vi "DSDLL Fetch From Digitizing Process.vi"(7 "max wait for packet [ms]":i32=50, 8 "error in":errorcluster, 11 "dsdll in":T3) -> (0 "error out":errorcluster, 1 "auxiliary sampling data":T1, 2 "data block":T2, 3 "dsdll out":T3, 4 "fetching done?":bool)   [LabVIEW 2013, in "DSDLL Virtual Digitizer.lvlib"]
doc: "Tries to fetch data block from digitizing data queue. It waits for predefined amount of time. If fetch timeout is reached it returns no data and no error. If digitizing or fetching timeout is reached it returns timout error. If the last data block was detected it also waits for digitizing process exit. If the process won't return it generates error. If the \ndigitizing process terminates prematurely it will return error. The 'auxiliary sampling data' are valid only if 'valid?' flag in it is True. 'Data block' content is valid only if 'valid?' flag is true. The caller of this VI must collect the data whenever the 'valid?' flag(s) are True. Caller of this VI must always check 'fetching done?' flag and when it is True or function returned error it shall not be called again."
uses:
  DSDLL Virtual Digitizer.lvlib
  DSDLL Session.ctl
  dsdll.lvlibp/dsdll_instance.ctl
  dsdll.lvlibp/dsdll_device_record.ctl
  DSDLL Process Config.ctl
  DSDLL Data Packet.ctl
  DSDLL Aux Record Data.ctl
  <vilib>/Utility/error.llb/Error Cluster From Error Code.vi
  <vilib>/ErrorRing/Error Ring.xnode
  dsdll.lvlibp
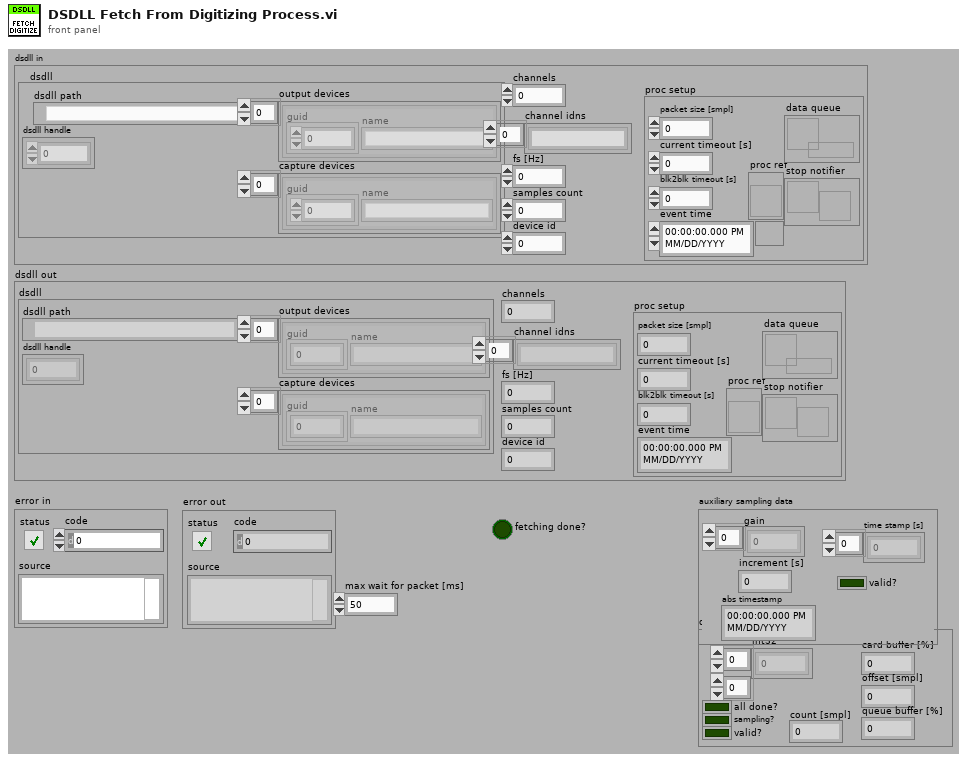
[diagram p1: front panel]
types:
  T1 = typedef "DSDLL Virtual Digitizer.lvlib/DSDLL Aux Record Data.ctl" = cluster{"time stamp [s]":dbl[], "gain":dbl[], "increment [s]":dbl, "valid?":bool, "abs timestamp":timestamp}
  T2 = typedef "DSDLL Virtual Digitizer.lvlib/DSDLL Data Packet.ctl" = cluster{"int32":i32[][], "card buffer [%]":dbl, "all done?":bool, "offset [smpl]":i32, "sampling?":bool, "queue buffer [%]":dbl, "count [smpl]":i32, "valid?":bool}
  T3 = typedef "DSDLL Virtual Digitizer.lvlib/DSDLL Session.ctl" = cluster{"dsdll":T4, "channels":i32, "device id":i32, "channel idns":string[], "proc setup":T6, "samples count":i32, "fs [Hz]":dbl}
  T4 = typedef "dsdll.lvlibp/dsdll_instance.ctl" = cluster{"dsdll path":path, "dsdll handle":u8[], "output devices":T5[], "capture devices":T5[]}
  T5 = typedef "dsdll.lvlibp/dsdll_device_record.ctl" = cluster{"guid":u8[], "name":string}
  T6 = typedef "DSDLL Virtual Digitizer.lvlib/DSDLL Process Config.ctl" = cluster{"packet size [smpl]":i32, "current timeout [s]":dbl, "blk2blk timeout [s]":dbl, "event time":timestamp, "data queue":refnum<queue>, "stop notifier":refnum<notifier>, "proc ref":refnum<vi>}
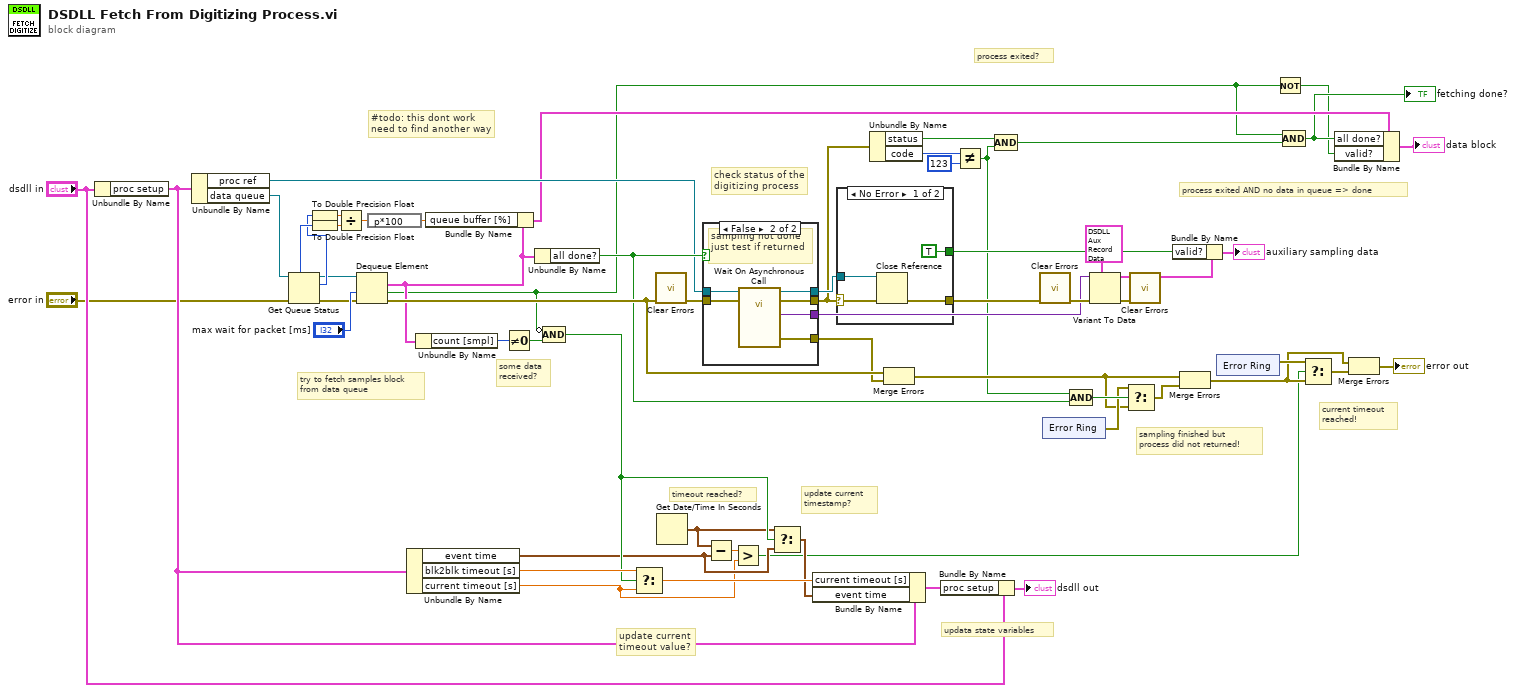
[diagram p0: block diagram]
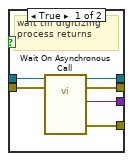
[diagram p3: hidden frame]
diagram:
  # "process exited AND no data in queue => done"
  # "process exited?"
  # "update current\ntimestamp?"
  # "update current \ntimeout value?"
  # "some data\nreceived?"
  # "#todo: this dont work\nneed to find another way"
  # "updata state variables"
  # "check status of the\ndigitizing process"
  # "try to fetch samples block\nfrom data queue"
  # "current timeout\nreached!"
  # "sampling finished but\nprocess did not returned!"
  # "timeout reached?"
  n1 = Unbundle By Name("dsdll in") -> ("proc setup"=w41:T6)
  n2 = Unbundle By Name(w41) -> ("proc ref"=w42:refnum<vi>, "data queue"=w29:refnum<queue>)
  n3 = Get Queue Status(queue=w29, error in (no error)="error in") -> (queue out=w31:refnum<queue>, max queue size=w37:i32, # pending remove=w32:i32, error out=w38:errorcluster)  [unwired: 1 in, 4 out]
  n4 = To Double Precision Float(number=w32) -> (double precision float=w33:dbl)
  n5 = To Double Precision Float(number=w37) -> (double precision float=w34:dbl)
  n6 = Divide(x=w33, y=w34) -> (x/y=w36:dbl)
  n7 = Dequeue Element(queue=w31, timeout in ms (-1)="max wait for packet [ms]", error in (no error)=w38) -> (element=w25:T2, timed out?=w1:bool, error out=w57:errorcluster)  [unwired: 1 out]
  n8 = expression code="p*100"(w36) -> (w35:dbl)
  n9 = Unbundle By Name(w41) -> ("event time"=w19:timestamp, "blk2blk timeout [s]"=w22:dbl, "current timeout [s]"=w3:dbl)
  n10 = Unbundle By Name(w25) -> ("count [smpl]"=w24:i32)
  n11 = Bundle By Name(cluster=w25, "queue buffer [%]"=w35) -> (w26:T2)
  n12 = Not Equal To 0?(x=w24) -> (x != 0?=w23:bool)
  n13 = Unbundle By Name(w25) -> ("all done?"=w49:bool)
  n14 = Compound Arithmetic op=AND(invert w1, w23) -> (w21:bool)
  n15 = Select(t=w22, s=w21, f=w3) -> (s? t:f=w18:dbl)
  n16 = call <vilib>:"Clear Errors.vi"("error in (no error)"=w57) -> ("error out"=w58:errorcluster)  [unwired: 6 in]
  n17 = Get Date/Time In Seconds() -> (seconds since 1Jan1904=w20:timestamp)
  n18 = case shown="False" w49 {
    tunnel: w42 -> [w66 w72]
    tunnel: w58 -> [w65 w71]
    tunnel: [w64 w70] -> w56
    tunnel: [w63 w69] -> w10
    tunnel: [w62 w68] -> w12
    tunnel: [w61 w67] -> w43
    frame True {
      # "wait till digitizing\nprocess returns"
      n19 = call-by-ref "Wait On Asynchronous Call"(reference=w66, error in=w65) -> (reference out=w61:refnum<vi>, error out=w63:errorcluster, 0:"error out"=w64:errorcluster, "auxiliary data out"=w62:variant)  [unwired: 10 in]
    }
    frame False {
      # "sampling not done\njust test if returned"
      n20 = call-by-ref "Wait On Asynchronous Call"(reference=w72, error in=w71) -> (reference out=w67:refnum<vi>, error out=w69:errorcluster, 0:"error out"=w70:errorcluster, "auxiliary data out"=w68:variant)  [unwired: 10 in]
    }
  }
  n21 = Subtract(x=w20, y=w19) -> (x-y=w59:dbl)
  n22 = Greater?(x=w59, y=w3) -> (0:w16:bool)
  n23 = Select(t=w20, s=w21, f=w19) -> (s? t:f=w17:timestamp)
  n24 = Bundle By Name(cluster=w41, "current timeout [s]"=w18, "event time"=w17) -> (w40:T6)
  n25 = case shown="No Error" w10 {
    selector: w10 -> [w76 w77]
    tunnel: [w75 w77] -> w44
    tunnel: w43 -> [w74 _]
    tunnel: [TRUE _] -> w11
    frame No Error {
      n26 = Close Reference(reference=w74, error in (no error)=w76) -> (error out=w75:errorcluster)
    }
    frame Error {
      # "timeout or\nalready eaxited"
    }
  }
  n27 = Unbundle By Name(w10) -> ("status"=w7:bool, "code"=w9:i32)
  n28 = Merge Errors(w57, w56) -> (w52:errorcluster)
  n29 = Bundle By Name(cluster="dsdll in", "proc setup"=w40) -> (→"dsdll out":T3)
  n30 = Not Equal?(x=w9, y=123) -> (x != y?=w2:bool)
  n31 = Compound Arithmetic op=AND(w7, w2) -> (w6:bool)
  n32 = call <vilib>:"Clear Errors.vi"("error in (no error)"=w44) -> ("error out"=w50:errorcluster)  [unwired: 6 in]
  n33 = xnode "Error Ring"() -> ("error out"=w53:errorcluster)
  n34 = Compound Arithmetic op=AND(w2, w49) -> (w54:bool)
  n35 = Variant To Data(error in=w50, type=T1 {"time stamp [s]"=[], "gain"=[], "increment [s]"=0.0, "valid?"=FALSE, "abs timestamp"=timestamp(0 s since 1904-01-01)} ("aux data"), Variant=w12) -> (data=w14:T1, error out=w13:errorcluster)
  n36 = Select(t=w53, s=w54, f=w52) -> (s? t:f=w51:errorcluster)
  n37 = call <vilib>:"Clear Errors.vi"("error in (no error)"=w13) -> ()  [unwired: 6 in, 1 out]
  n38 = Bundle By Name(cluster=w14, "valid?"=w11) -> (→"auxiliary sampling data":T1)
  n39 = Merge Errors(w52, w51) -> (w46:errorcluster)
  n40 = xnode "Error Ring"() -> ("error out"=w48:errorcluster)
  n41 = Not(x=w1) -> (.not. x?=w4:bool)
  n42 = Compound Arithmetic op=AND(w1, w6) -> (w5:bool)
  "fetching done?" <- w5
  n43 = Select(t=w48, s=w16, f=w46) -> (s? t:f=w47:errorcluster)
  n44 = Bundle By Name(cluster=w26, "all done?"=w5, "valid?"=w4) -> (→"data block":T2)
  n45 = Merge Errors(w46, w47) -> (→"error out":errorcluster)
